vi "terminal voltage readbacks.vi"() -> ()   [LabVIEW 2016]
doc: "This vi uses the control room rio to readback the terminal voltage settings. It must have the control room rio in the project to run correctly"
panel:
  out "sum":dbl format="%#.3g"
  out "Grid":dbl format="%#.3g"
  out "error out":errorcluster
  in  "stop":bool
  out "Le Chain":dbl format="%#.3g"
  out "Le Column":dbl format="%#.3g"
  out "Le IND":dbl format="%.2f"
  out "LE Supp":dbl format="%.2f"
  out "He Chain":dbl format="%#.3g"
  out "HE Column":dbl format="%#.2g"
  out "He ind":dbl format="%.2f"
  out "He Supp":dbl format="%#.5g"
  out "Corona Current":dbl format="%#.3g"
  out "Terminal voltage":dbl format="%#.3g"
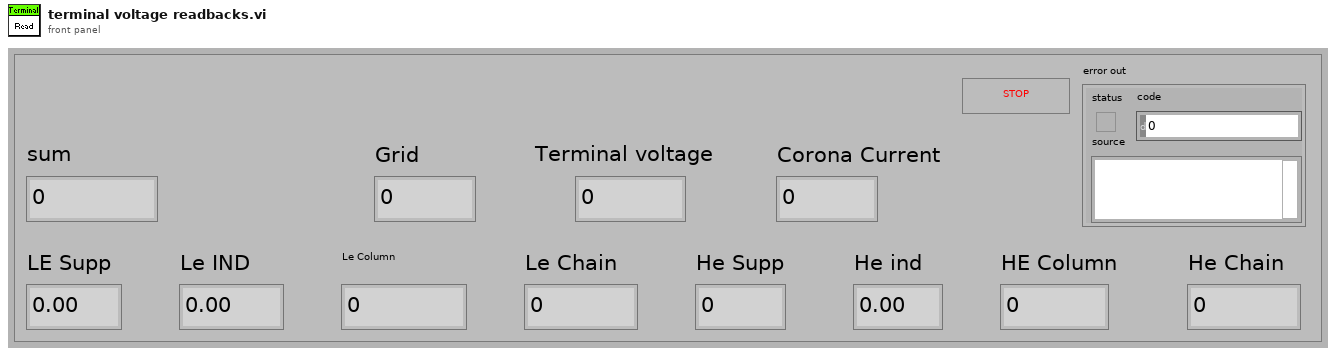
[diagram p1: front panel]
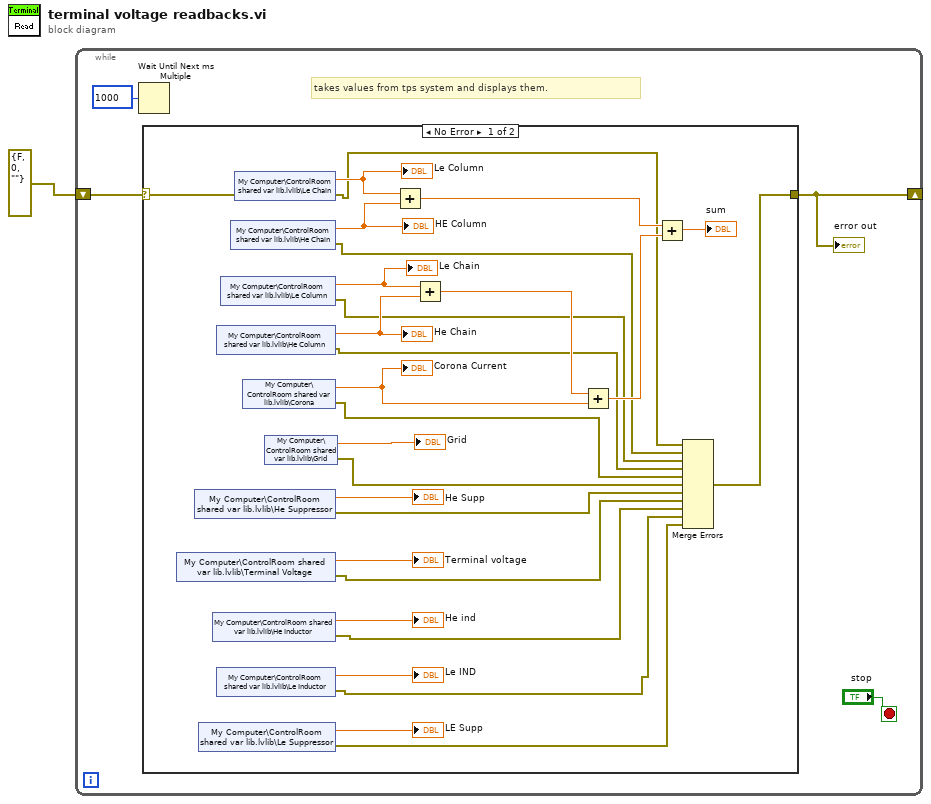
[diagram p0: block diagram]
diagram:
  n1 = while {
    shift-right: [w2] -> _
    shift-left: errorcluster {"status"=FALSE, "code"=0, "source"=""} ("error in (no error)") -> [w3]
    stop <- "stop" stop-if-true
    # "takes values from tps system and displays them."
    n2 = Wait Until Next ms Multiple(millisecond multiple=u32 1000) -> ()  [unwired: 1 out]
    n3 = case shown="No Error" w3 {
      selector: w3 -> [w18 w34]
      tunnel: [w16 w34] -> w2
      frame No Error {
        n4 = shared-variable "My Computer\\ControlRoom shared var lib.lvlib\\Terminal Voltage"() -> (→"Terminal voltage":dbl, error out=w13:errorcluster)  [unwired: 1 in]
        n5 = shared-variable "My Computer\\ControlRoom shared var lib.lvlib\\He Suppressor"() -> (→"He Supp":dbl, error out=w12:errorcluster)  [unwired: 1 in]
        n6 = shared-variable "My Computer\\ControlRoom shared var lib.lvlib\\Le Suppressor"() -> (→"LE Supp":dbl, error out=w17:errorcluster)  [unwired: 1 in]
        n7 = shared-variable "My Computer\\ControlRoom shared var lib.lvlib\\He Inductor"() -> (→"He ind":dbl, error out=w14:errorcluster)  [unwired: 1 in]
        n8 = shared-variable "My Computer\\ControlRoom shared var lib.lvlib\\He Column"() -> (w25:dbl, error out=w9:errorcluster)  [unwired: 1 in]
        "He Chain" <- w25
        n9 = shared-variable "My Computer\\ControlRoom shared var lib.lvlib\\Le Inductor"() -> (→"Le IND":dbl, error out=w15:errorcluster)  [unwired: 1 in]
        n10 = shared-variable "My Computer\\ControlRoom shared var lib.lvlib\\Le Column"() -> (w19:dbl, error out=w8:errorcluster)  [unwired: 1 in]
        "Le Chain" <- w19
        n11 = shared-variable "My Computer\\ControlRoom shared var lib.lvlib\\He Chain"() -> (w20:dbl, error out=w7:errorcluster)  [unwired: 1 in]
        "HE Column" <- w20
        n12 = shared-variable "My Computer\\ControlRoom shared var lib.lvlib\\Le Chain"(error in=w18) -> (w30:dbl, error out=w6:errorcluster)
        "Le Column" <- w30
        n13 = shared-variable "My Computer\\ControlRoom shared var lib.lvlib\\Corona"() -> (w24:dbl, error out=w10:errorcluster)  [unwired: 1 in]
        "Corona Current" <- w24
        n14 = shared-variable "My Computer\\ControlRoom shared var lib.lvlib\\Grid"() -> (→"Grid":dbl, error out=w11:errorcluster)  [unwired: 1 in]
        n15 = Add(x=w30, y=w20) -> (x+y=w21:dbl)
        n16 = Add(x=w19, y=w25) -> (x+y=w23:dbl)
        n17 = Add(x=w23, y=w24) -> (x+y=w22:dbl)
        n18 = Add(x=w21, y=w22) -> (x+y=→"sum":dbl)
        n19 = Merge Errors(w6, w7, w8, w9, w10, w11, w12, w13, w14, w15, w17) -> (w16:errorcluster)
      }
      frame Error {
      }
    }
    "error out" <- w2
  }
